vi "IMAQ FPGA Camera Link Line Builder (2 Tap U8 2X-1Y).vi"(8 "Input Valid In":bool=TRUE, 9 "Frame Valid In":bool, 10 "Line Valid In":bool, 11 "Pixel Data In":u8[](array[numeric])=[0, 0]) -> (0 "Output Valid":bool, 1 "Frame Valid Out":bool, 2 "Line Valid Out":bool, 3 "Pixel Bus x8 Out":cluster{"Pixels":u8[], "DV":bool[]}, 5 "Overflow":bool)   [LabVIEW 2020]
doc: "Camera Link cameras may return pixels from different parts of the image on each pixel clock. The Line Builder takes those pixels and combines them over multiple cycles to return a Pixel Bus of 8 pixels that are adjacent to each other. \n\nThis instance expects a camera with two taps (i.e. two pixels returned on each pixel clock). The first tap represents the left half of the image and the first valid pixels from this tap is located on the left of the image (pixels 0). The next tap represents the right half of the image and the first valid pixel from this tap is located at the center of the image."
uses:
  <vilib>/visionFPGA/Basics/Camera Link Acquisition/Controls/IMAQ FPGA Camera Link Line Builder State.ctl
  <vilib>/rvi/Emulation/niFpgaSctlEmulationGetInTimedLoop.vi
  <vilib>/Utility/error.llb/Clear Errors.vi
  <vilib>/rvi/DataTransferAndStorage/Container/Common/niFpgaContainerGetUniqueNameForEmu.vi
  <vilib>/rvi/DataTransferAndStorage/Container/Common/niFpgaContainerSetEmuInfo.vi
  <vilib>/rvi/eio/common/nirviEmuReportErrorAndStop.vi
  <vilib>/rvi/DataTransferAndStorage/Container/Common/niFpgaContainerExecOnDevCompGetState.vi
  <vilib>/rvi/Emulation/niFpgaEmulationIsFPGAContextNoSignature.vi
  <vilib>/rvi/Emulation/niFpgaProcessEmulError.vi
  <vilib>/rvi/errors/nirviReportUnexpectedCaseInternalError (U32).vi
  <vilib>/rvi/Memory/Memory_Emulation/niFpgaMemoryEmulationCacheClearOnFirstRun.vi
  <vilib>/rvi/Memory/Memory_Emulation/nirvimemoryEmulationManagerCache_MakeExclusive.vi
  <vilib>/rvi/Memory/Memory_Emulation/niFpgaMemoryEmulationValidateCache.vi
  <vilib>/rvi/Memory/Memory_Emulation/nirvimemoryEmulationManagerCache_InsertValue.vi
  <vilib>/rvi/Memory/Memory_Emulation/nirvimemoryEmulationManagerCache_ReleaseExclusive.vi
  <vilib>/rvi/Memory/Memory_Emulation/nirvimemoryEmulationManagerCache_GetValue.vi
  <vilib>/rvi/Memory/Memory_Emulation/nirvimemoryEmulationManagerCache_SetValue.vi
  <vilib>/rvi/Emulation/niFpgaSctlEmulationResourceMgr.vi
  <vilib>/rvi/LocalResourceManager/LocalResourceManager.xnode
  <vilib>/rvi/DataTransferAndStorage/Container/XNode/niFpgaContainer.xnode
  <vilib>/rvi/Memory/Memory_Emulation/niFpgaMemoryEmulationRefIn.vi
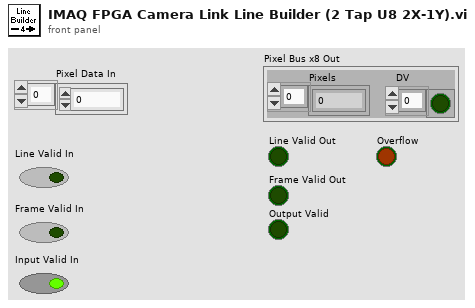
[diagram p1: front panel]
types:
  T1 = typedef "IMAQ FPGA Camera Link Line Builder State.ctl" = enum16{"Wait for First Valid Pixels", "Update Section 1", "Update Section 2", "Update Section 3", "Update Last Section", "Add Final Pack", "Add End of Line", "Check End of Image"}
  T2 = cluster{bool, u16, "Falling Edge":bool, bool, "Falling Edge":bool}
  T3 = cluster{bool, u16, "Falling Edge":bool, "Enum":T1, "Falling Edge":bool}
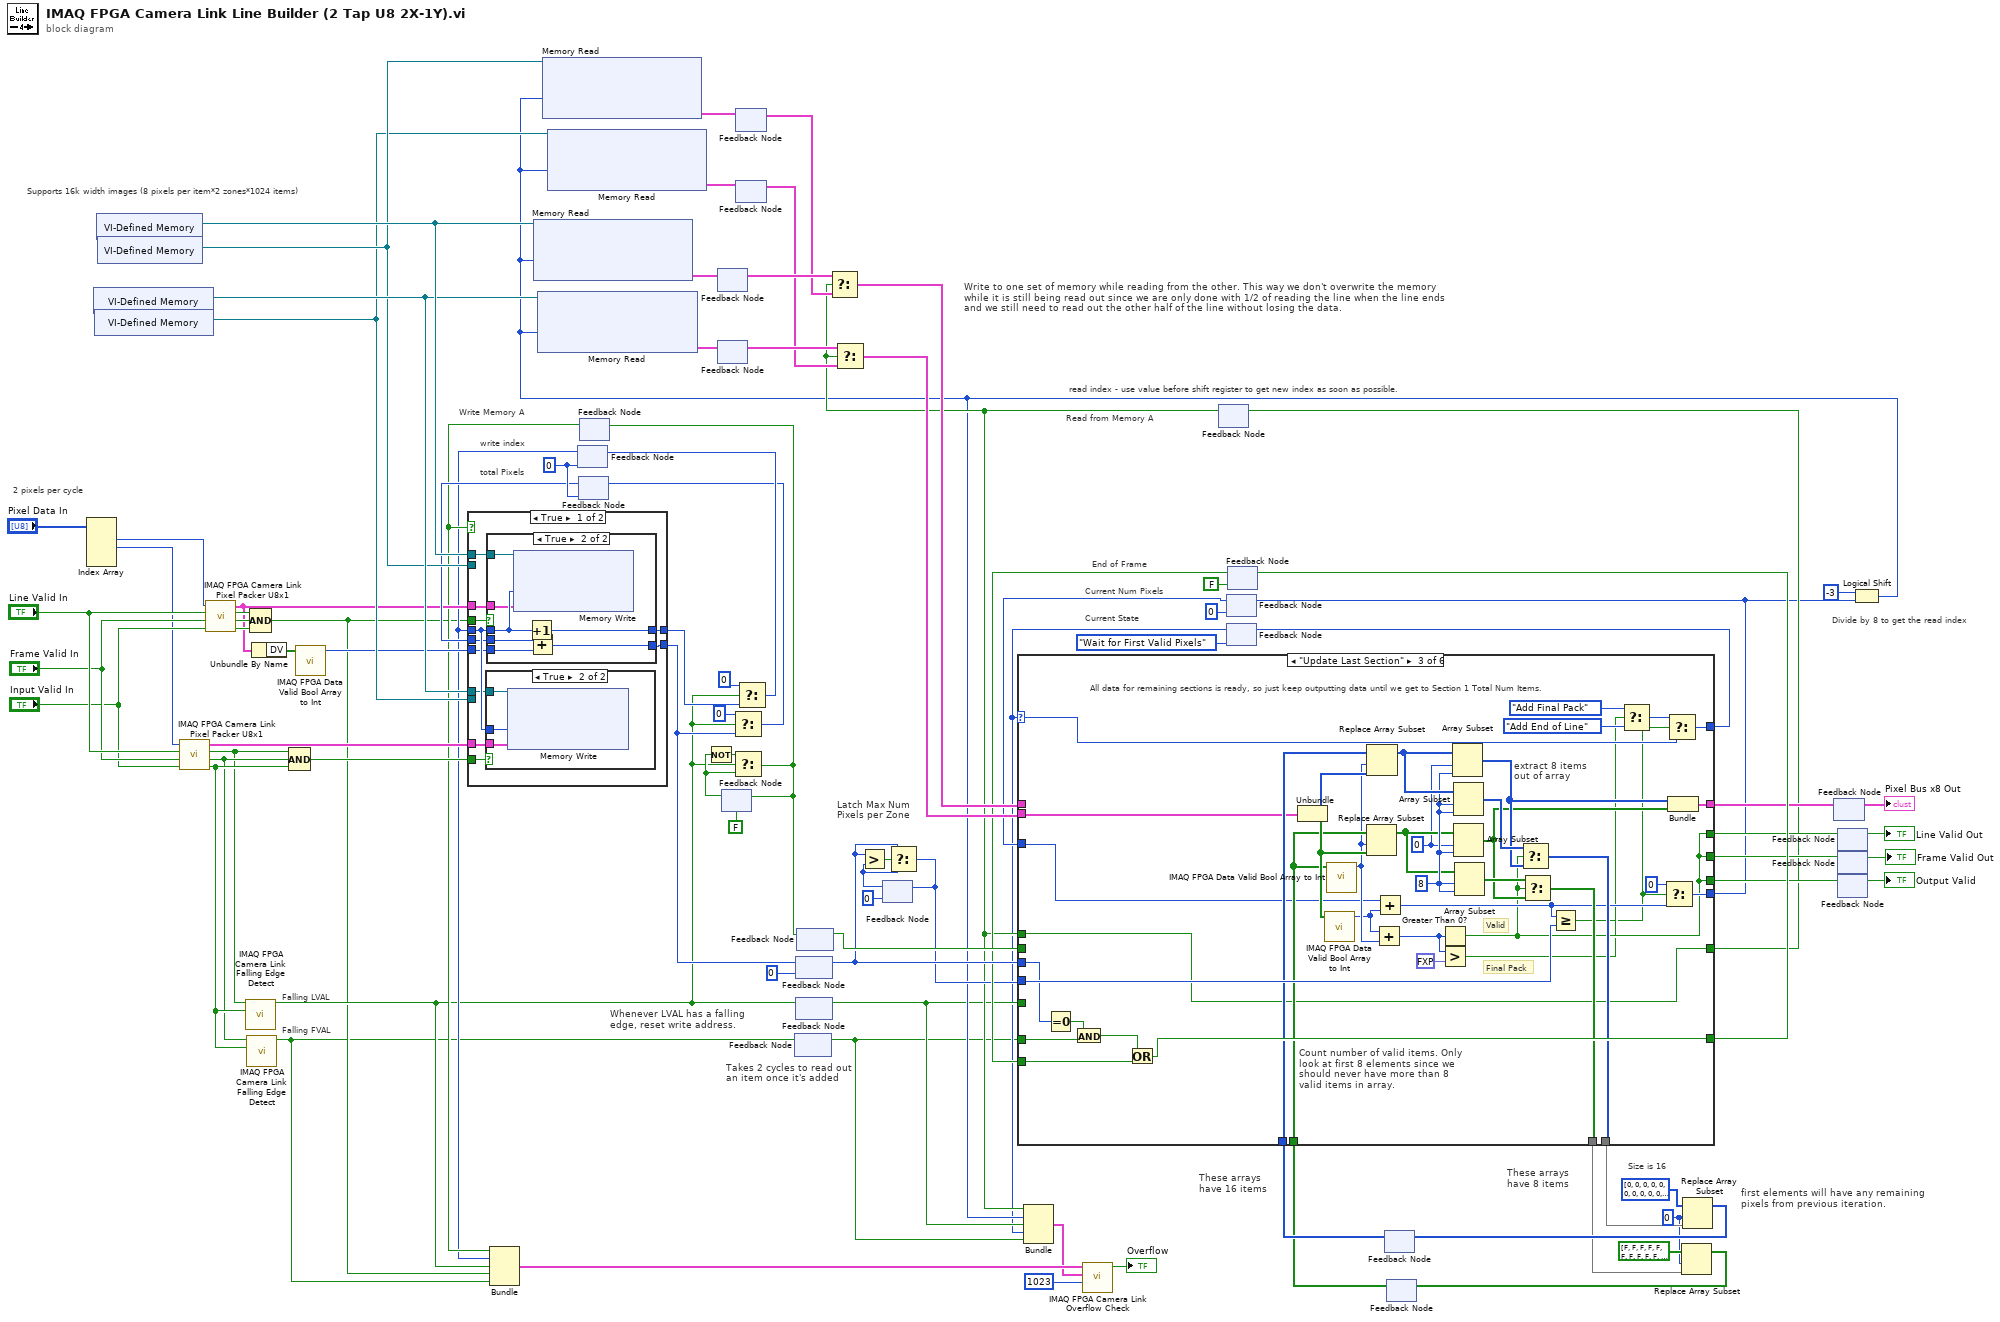
[diagram p0: block diagram]
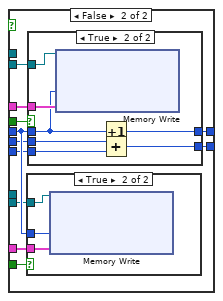
[diagram p4: hidden frame]
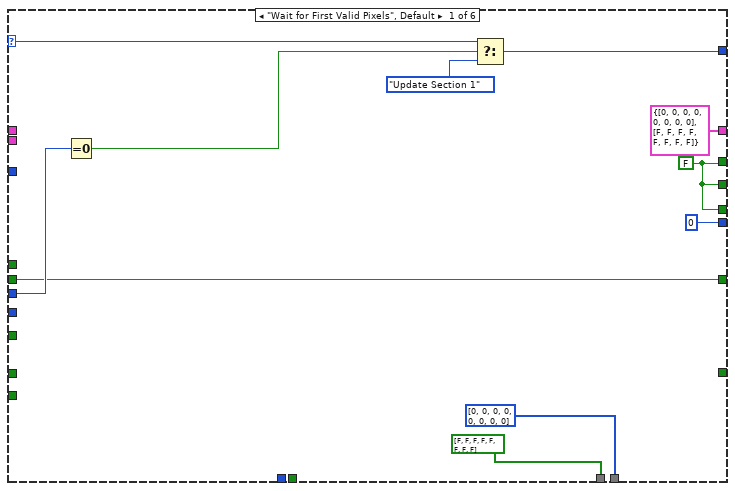
[diagram p7: hidden frame]
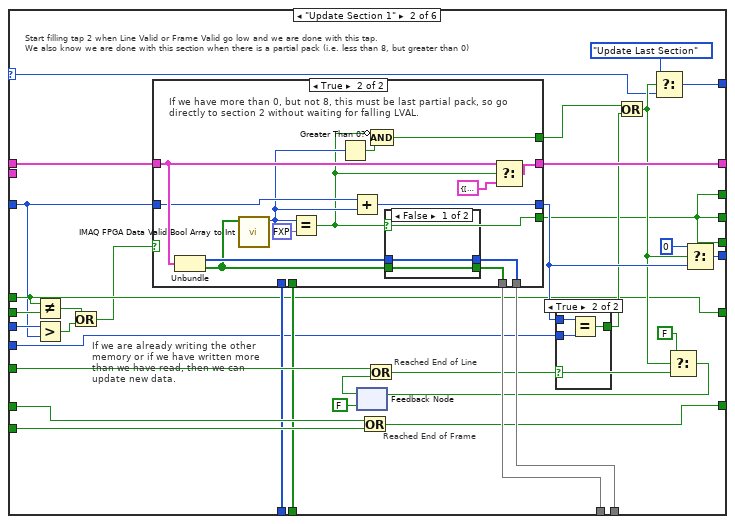
[diagram p8: hidden frame]
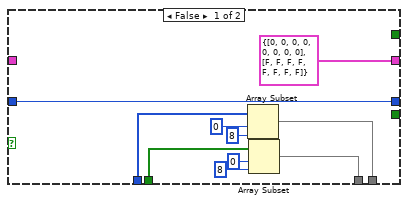
[diagram p9: hidden frame]
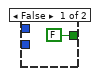
[diagram p11: hidden frame]
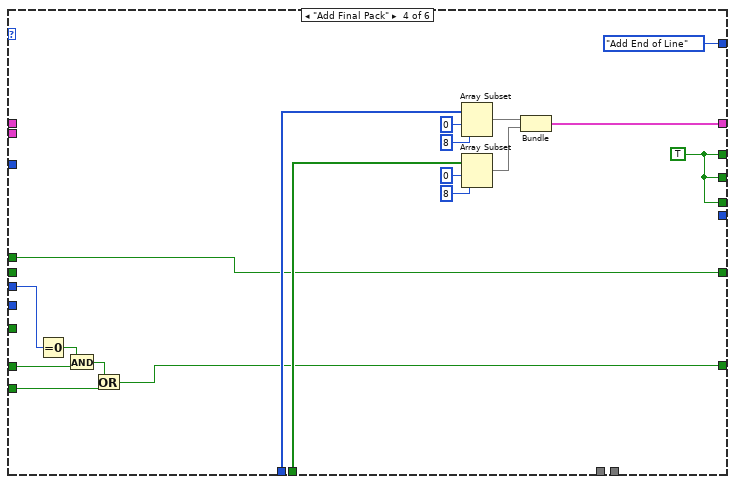
[diagram p12: hidden frame]
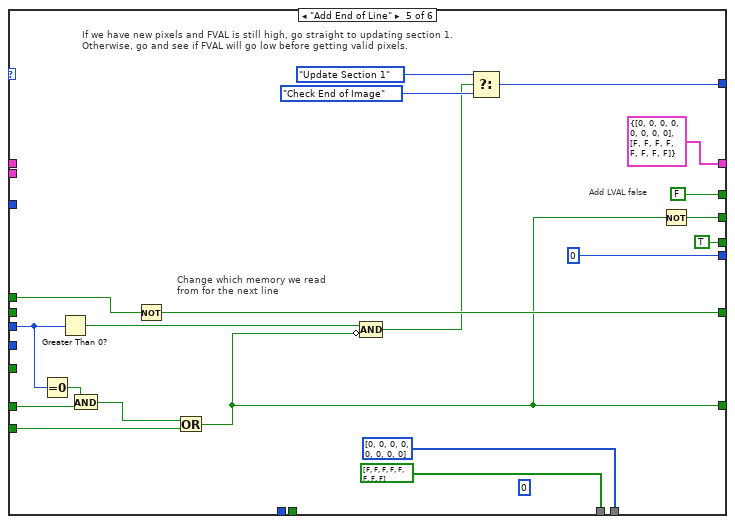
[diagram p13: hidden frame]
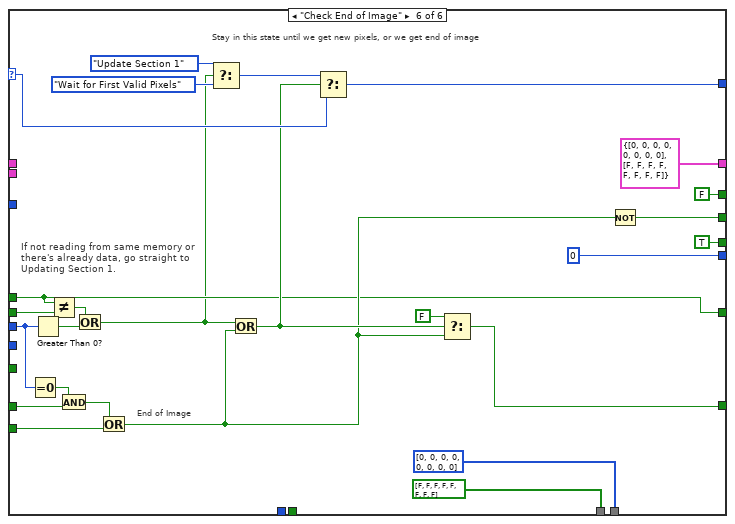
[diagram p14: hidden frame]
diagram:
  w43 = 0 ("index")
  w39 = u16 0
  # "Divide by 8 to get the read index"
  # "Latch Max Num Pixels per Zone"
  # "total Pixels"
  # "These arrays have 8 items"
  # "These arrays have 16 items"
  # "first elements will have any remaining pixels from previous iteration."
  # "Size is 16"
  # "Read from Memory A"
  # "Write Memory A"
  # "Write to one set of memory while reading from the other. This way we don't overwrite the memory while it is still being read out since we are only done with 1/2 of reading the line when the line ends and we still need to read out the other half of the line without losing the data."
  # "Falling FVAL"
  # "Falling LVAL"
  # "read index - use value before shift register to get new index as soon as possible."
  # "write index"
  # "Current State"
  # "End of Frame"
  # "Takes 2 cycles to read out an item once it's added"
  # "Current Num Pixels"
  # "Whenever LVAL has a falling edge, reset write address."
  # "Supports 16k width images (8 pixels per item*2 zones*1024 items)"
  # "2 pixels per cycle"
  n1 = Index Array(array="Pixel Data In") -> (element #1=w5:u8, element #2=w4:u8)  [unwired: 4 in, 2 out]
  n2 = xnode "VI-Defined Memory"() -> ("Memory Out"=w68:refnum<k21>)
  n3 = xnode "VI-Defined Memory"() -> ("Memory Out"=w64:refnum<k21>)
  n4 = xnode "VI-Defined Memory"() -> ("Memory Out"=w69:refnum<k21>)
  n5 = xnode "VI-Defined Memory"() -> ("Memory Out"=w65:refnum<k21>)
  n6 = call <vilib>:"IMAQ FPGA Camera Link Pixel Packer U8x1.vi"("Input Valid"="Input Valid In", "Frame Valid In"="Frame Valid In", "Line Valid In"="Line Valid In", "Pixel In"=w4) -> ("Output Valid"=w3:bool, "Frame Valid Out"=w2:bool, "Line Valid Out"=w1:bool, "Pixel Bus x8 Out"=w57:cluster{"Pixels":u8[], "DV":bool[]})  [unwired: 4 in]
  n7 = call <vilib>:"IMAQ FPGA Camera Link Pixel Packer U8x1.vi"("Input Valid"="Input Valid In", "Frame Valid In"="Frame Valid In", "Line Valid In"="Line Valid In", "Pixel In"=w5) -> ("Output Valid"=w83:bool, "Frame Valid Out"=w84:bool, "Line Valid Out"=w85:bool, "Pixel Bus x8 Out"=w33:cluster{"Pixels":u8[], "DV":bool[]})  [unwired: 4 in]
  n8 = call <vilib>:"IMAQ FPGA Camera Link Falling Edge Detect.vi"("Input Valid"=w3, "Input"=w1) -> ("Falling Edge"=w17:bool)  [unwired: 9 in]
  n9 = call <vilib>:"IMAQ FPGA Camera Link Falling Edge Detect.vi"("Input Valid"=w3, "Input"=w2) -> ("Falling Edge"=w15:bool)  [unwired: 9 in]
  n10 = Compound Arithmetic op=AND(w85, w84, w83) -> (w16:bool)
  n11 = Unbundle By Name(w33) -> ("DV"=w42:bool[])
  n12 = Compound Arithmetic op=AND(w1, w2, w3) -> (w55:bool)
  n13 = call <vilib>:"IMAQ FPGA Data Valid Bool Array to Int.vi"("DV In"=w42) -> ("Sum DV Out"=w37:u8)  [unwired: 10 in]
  n14 = feedback #1(w39) -> (w18:u16)
  n15 = feedback #2(w39) -> (w38:u16)
  n16 = feedback #3() -> (w19:bool)  [unwired: 1 in]
  n17 = case shown="True" w19 {
    tunnel: [w102 w125] -> w86
    tunnel: w18 -> [w101 w124]
    tunnel: w16 -> [w96 w123]
    tunnel: w33 -> [w100 w122]
    tunnel: w57 -> [w99 w121]
    tunnel: w69 -> [w98 _]
    tunnel: w68 -> [w97 _]
    tunnel: w65 -> [_ w120]
    tunnel: w64 -> [_ w119]
    tunnel: w55 -> [w95 w118]
    tunnel: [w94 w117] -> w36
    tunnel: w38 -> [w93 w116]
    tunnel: w37 -> [w92 w115]
    frame True {
      n18 = case shown="True" w95 {
        tunnel: w99 -> [_ w104]
        tunnel: w97 -> [_ w105]
        tunnel: w101 -> [_ w103]
        frame False {
        }
        frame True {
          n19 = xnode ("Memory Write")("Address"=w103, "Data"=w104, "Memory In"=w105) -> ()  [unwired: 1 out]
        }
      }
      n20 = case shown="True" w96 {
        tunnel: [w106 w108] -> w102
        tunnel: w101 -> [w107 w113]
        tunnel: w98 -> [_ w114]
        tunnel: w100 -> [_ w112]
        tunnel: [w107 w111] -> w94
        tunnel: w93 -> [w106 w110]
        tunnel: w92 -> [_ w109]
        frame False {
        }
        frame True {
          n21 = xnode ("Memory Write")("Address"=w113, "Data"=w112, "Memory In"=w114) -> ()  [unwired: 1 out]
          n22 = Increment(x=w113) -> (x+1=w111:u16)
          n23 = Add(x=w110, y=w109) -> (x+y=w108:u16)
        }
      }
    }
    frame False {
      n24 = case shown="True" w118 {
        tunnel: w121 -> [_ w127]
        tunnel: w119 -> [_ w128]
        tunnel: w124 -> [_ w126]
        frame False {
        }
        frame True {
          n25 = xnode ("Memory Write")("Address"=w126, "Data"=w127, "Memory In"=w128) -> ()  [unwired: 1 out]
        }
      }
      n26 = case shown="True" w123 {
        tunnel: [w129 w133] -> w125
        tunnel: w124 -> [w130 w135]
        tunnel: w120 -> [_ w137]
        tunnel: w122 -> [_ w136]
        tunnel: [w130 w134] -> w117
        tunnel: w116 -> [w129 w132]
        tunnel: w115 -> [_ w131]
        frame False {
        }
        frame True {
          n27 = xnode ("Memory Write")("Address"=w135, "Data"=w136, "Memory In"=w137) -> ()  [unwired: 1 out]
          n28 = Increment(x=w135) -> (x+1=w134:u16)
          n29 = Add(x=w132, y=w131) -> (x+y=w133:u16)
        }
      }
    }
  }
  n30 = Bundle(w19, w18, "Falling Edge"=w17, w16, "Falling Edge"=w15) -> (w14:T2)  [unwired: 1 in]
  n31 = feedback #4() -> (w61:cluster{"Pixels":u8[], "DV":bool[]})  [unwired: 1 in]
  n32 = feedback #5() -> (w59:cluster{"Pixels":u8[], "DV":bool[]})  [unwired: 1 in]
  n33 = feedback #6(FALSE) -> (w41:bool)
  n34 = Not(x=w41) -> (.not. x?=w81:bool)
  n35 = Select(t=u16 0, s=w17, f=w86) -> (s? t:f=w34:u16)
  n36 = feedback-in #2(w34) -> ()
  n37 = Select(t=w81, s=w17, f=w41) -> (s? t:f=w32:bool)
  n38 = feedback-in #3(w32) -> ()
  n39 = feedback-in #6(w32) -> ()
  n40 = feedback #7() -> (w60:cluster{"Pixels":u8[], "DV":bool[]})  [unwired: 1 in]
  n41 = feedback #8() -> (w58:cluster{"Pixels":u8[], "DV":bool[]})  [unwired: 1 in]
  n42 = Select(t=u16 0, s=w17, f=w36) -> (s? t:f=w35:u16)
  n43 = feedback-in #1(w35) -> ()
  n44 = feedback #9() -> (w8:bool)  [unwired: 1 in]
  n45 = feedback-in #9(w15) -> ()
  n46 = feedback-in #10(w86) -> ()
  n47 = feedback #10(u16 0) -> (w30:u16)
  n48 = feedback-in #11(w17) -> ()
  n49 = feedback #11() -> (w11:bool)  [unwired: 1 in]
  n50 = feedback #12() -> (w47:bool)  [unwired: 1 in]
  n51 = feedback-in #12(w32) -> ()
  n52 = feedback #13(u16 0) -> (w29:u16)
  n53 = Greater?(x=w30, y=w29) -> (0:w31:bool)
  n54 = Select(t=w30, s=w31, f=w29) -> (s? t:f=w20:u16)
  n55 = feedback-in #13(w20) -> ()
  n56 = feedback #14() -> (w13:bool)  [unwired: 1 in]
  n57 = Select(t=w61, s=w13, f=w60) -> (s? t:f=w46:cluster{"Pixels":u8[], "DV":bool[]})
  n58 = Select(t=w59, s=w13, f=w58) -> (s? t:f=w56:cluster{"Pixels":u8[], "DV":bool[]})
  n59 = feedback #15(u16 0) -> (w22:u16)
  n60 = feedback #16(IMAQ_FPGA_Camera_Link_Line_Builder_State."Wait for First Valid Pixels" ("Enum")) -> (w9:T1)
  n61 = feedback #17(FALSE) -> (w24:bool)
  n62 = feedback #18() -> (w45:u8[])  [unwired: 1 in]
  n63 = feedback #19() -> (w44:bool[])  [unwired: 1 in]
  n64 = case shown="\"Update Last Section\"" w9 {
    selector: w9 -> [w148 w149 w239 _ _ w309]
    tunnel: [w147 w181 w251 IMAQ_FPGA_Camera_Link_Line_Builder_State."Add End of Line" ("Enum") w284 w310] -> w21
    tunnel: w11 -> [_ w179 _ _ _ _]
    tunnel: w8 -> [_ w175 w221 w253 w273 w296]
    tunnel: [u16 0 w178 w247 _ u16 0 u16 0] -> w27
    tunnel: w22 -> [_ w155 w228 _ _ _]
    tunnel: w30 -> [w143 w156 w222 w254 w274 w297]
    tunnel: w20 -> [_ w168 w248 _ _ _]
    tunnel: [_ w171 w249 w256 w270 w306] -> w87
    tunnel: w24 -> [_ w176 w250 w257 w288 w312]
    tunnel: w46 -> [_ w165 _ _ _ _]
    tunnel: w56 -> [_ _ w214 _ _ _]
    tunnel: w47 -> [w142 w158 _ _ _ w293]
    tunnel: [w142 w159 w216 w258 w279 w292] -> w48
    tunnel: w13 -> [_ w159 w216 w258 w280 w292]
    tunnel: w44 -> [_ w169 w238 w261 _ _]
    tunnel: w45 -> [_ w170 w243 w262 _ _]
    tunnel: [cluster{"Pixels":u8[], "DV":bool[]} {"Pixels"=[0, 0, 0, 0, 0, 0, 0, 0], "DV"=[FALSE, FALSE, FALSE, FALSE, FALSE, FALSE, FALSE, FALSE]} ("Data") w174 w246 w260 cluster{"Pixels":u8[], "DV":bool[]} {"Pixels"=[0, 0, 0, 0, 0, 0, 0, 0], "DV"=[FALSE, FALSE, FALSE, FALSE, FALSE, FALSE, FALSE, FALSE]} ("Data") cluster{"Pixels":u8[], "DV":bool[]} {"Pixels"=[0, 0, 0, 0, 0, 0, 0, 0], "DV"=[FALSE, FALSE, FALSE, FALSE, FALSE, FALSE, FALSE, FALSE]} ("Data")] -> w77
    tunnel: [w138 w152 w219 w259 FALSE FALSE] -> w75
    tunnel: [w138 w152 w219 w259 w281 w302] -> w74
    tunnel: [w138 w152 w219 w259 TRUE TRUE] -> w73
    tunnel: [bool[] [FALSE, FALSE, FALSE, FALSE, FALSE, FALSE, FALSE, FALSE] ("DV") w173 w232 _ bool[] [FALSE, FALSE, FALSE, FALSE, FALSE, FALSE, FALSE, FALSE] bool[] [FALSE, FALSE, FALSE, FALSE, FALSE, FALSE, FALSE, FALSE]] -> w49
    tunnel: [u8[] [0, 0, 0, 0, 0, 0, 0, 0] ("Pixels") w172 w231 _ u8[] [0, 0, 0, 0, 0, 0, 0, 0] ("Pixels") u8[] [0, 0, 0, 0, 0, 0, 0, 0] ("Pixels")] -> w50
    frame "Wait for First Valid Pixels", Default {
      w138 = FALSE
      n65 = Equal To 0?(x=w143) -> (x = 0?=w146:bool)
      n66 = Select(t=w148, s=w146, f=IMAQ_FPGA_Camera_Link_Line_Builder_State."Update Section 1") -> (s? t:f=w147:T1)
    }
    frame "Update Section 1" {
      # "If we are already writing the other memory or if we have written more than we have read, then we can update new data."
      # "Reached End of Frame"
      # "Reached End of Line"
      # "Start filling tap 2 when Line Valid or Frame Valid go low and we are done with this tap.\nWe also know we are done with this section when there is a partial pack (i.e. less than 8, but greater than 0)"
      n67 = Not Equal?(x=w159, y=w158) -> (x != y?=w157:bool)
      n68 = Greater?(x=w156, y=w155) -> (0:w154:bool)
      n69 = Or(x=w157, y=w154) -> (x .or. y?=w153:bool)
      n70 = case shown="True" w153 {
        tunnel: w165 -> [_ w202]
        tunnel: w155 -> [w191 w200]
        tunnel: [w191 w205] -> w177
        tunnel: [cluster{"Pixels":u8[], bool[]} {"Pixels"=[0, 0, 0, 0, 0, 0, 0, 0], [FALSE, FALSE, FALSE, FALSE, FALSE, FALSE, FALSE, FALSE]} w204] -> w174
        tunnel: [w182 w195] -> w173
        tunnel: [w186 w196] -> w172
        tunnel: w170 -> [w189 _]
        tunnel: w169 -> [w185 _]
        tunnel: [_ w194] -> w152
        tunnel: [_ w192] -> w151
        frame False {
          n71 = Array Subset(array=w189, index=0, length=8) -> (w186:u8[])
          n72 = Array Subset(array=w185, index=0, length=8) -> (w182:bool[])
        }
        frame True {
          # "If we have more than 0, but not 8, this must be last partial pack, so go directly to section 2 without waiting for falling LVAL."
          n73 = Unbundle(w202) -> ("Pixels"=w198:u8[], "DV"=w197:bool[])
          n74 = call <vilib>:"IMAQ FPGA Data Valid Bool Array to Int.vi"("DV In"=w197) -> ("Sum DV Out"=w199:u8)  [unwired: 10 in]
          n75 = Equal?(x=w199, y=fxp<+,4,4> 8.0) -> (x = y?=w194:bool)
          n76 = Greater Than 0?(x=w199) -> (x > 0?=w193:bool)
          n77 = Add(x=w200, y=w199) -> (x+y=w205:u16)
          n78 = Compound Arithmetic op=AND(invert w194, w193) -> (w192:bool)
          n79 = case shown="False" w194 {
            tunnel: w198 -> [w207 _]
            tunnel: w197 -> [w206 _]
            tunnel: [w207 _] -> w196
            tunnel: [w206 _] -> w195
            frame False {
            }
            frame True {
            }
          }
          n80 = Select(t=w202, s=w194, f=cluster{"Pixels":u8[], "DV":bool[]} {"Pixels"=[0, 0, 0, 0, 0, 0, 0, 0], "DV"=[FALSE, FALSE, FALSE, FALSE, FALSE, FALSE, FALSE, FALSE]}) -> (s? t:f=w204:cluster{"Pixels":u8[], "DV":bool[]})
        }
      }
      n81 = feedback #20(FALSE) -> (w164:bool)
      n82 = Or(x=w175, y=w176) -> (x .or. y?=w171:bool)
      n83 = Or(x=w179, y=w164) -> (x .or. y?=w163:bool)
      n84 = case shown="True" w163 {
        tunnel: w168 -> [_ w210]
        tunnel: w177 -> [_ w211]
        tunnel: [FALSE w209] -> w166
        frame False {
        }
        frame True {
          n85 = Equal?(x=w211, y=w210) -> (x = y?=w209:bool)
        }
      }
      n86 = Or(x=w151, y=w166) -> (x .or. y?=w162:bool)
      n87 = Select(t=IMAQ_FPGA_Camera_Link_Line_Builder_State."Update Last Section" ("Enum"), s=w162, f=w149) -> (s? t:f=w181:T1)
      n88 = Select(t=FALSE, s=w162, f=w163) -> (s? t:f=w160:bool)
      n89 = feedback-in #20(w160) -> ()
      n90 = Select(t=u16 0, s=w162, f=w177) -> (s? t:f=w178:u16)
    }
    frame "Update Last Section" {
      w230 = 0 ("index")
      w241 = 8 ("length")
      # "Final Pack"
      # "Valid"
      # "extract 8 items out of array"
      # "Count number of valid items. Only look at first 8 elements since we should never have more than 8 valid items in array."
      # "All data for remaining sections is ready, so just keep outputting data until we get to Section 1 Total Num Items."
      n91 = Equal To 0?(x=w222) -> (x = 0?=w223:bool)
      n92 = And(x=w223, y=w221) -> (x .and. y?=w220:bool)
      n93 = Or(x=w220, y=w250) -> (x .or. y?=w249:bool)
      n94 = Unbundle(w214) -> ("Pixels"=w245:u8[], "DV"=w244:bool[])
      n95 = call <vilib>:"IMAQ FPGA Data Valid Bool Array to Int.vi"("DV In"=w244) -> ("Sum DV Out"=w227:u8)  [unwired: 10 in]
      n96 = call <vilib>:"IMAQ FPGA Data Valid Bool Array to Int.vi"("DV In"=w238) -> ("Sum DV Out"=w237:u8)  [unwired: 10 in]
      n97 = Replace Array Subset(array=w238, new element=w244, index=w237) -> (w240:bool[])
      n98 = Replace Array Subset(array=w243, new element=w245, index=w237) -> (w242:u8[])
      n99 = Add(x=w227, y=w237) -> (x+y=w217:u8)
      n100 = Add(x=w228, y=w227) -> (x+y=w229:u16)
      n101 = Greater Than 0?(x=w217) -> (x > 0?=w219:bool)
      n102 = Greater?(x=w217, y=fxp<+,5,5> 8.0) -> (0:w218:bool)
      n103 = Array Subset(array=w242, index=w230, length=w241) -> (w235:u8[])
      n104 = Array Subset(array=w242, index=w241, length=w241) -> (w236:u8[])
      n105 = Array Subset(array=w240, index=w230, length=w241) -> (w233:bool[])
      n106 = Array Subset(array=w240, index=w241, length=w241) -> (w234:bool[])
      n107 = Select(t=w236, s=w219, f=w235) -> (s? t:f=w231:u8[])
      n108 = Select(t=w234, s=w219, f=w233) -> (s? t:f=w232:bool[])
      n109 = Greater Or Equal?(x=w229, y=w248) -> (x >= y?=w212:bool)
      n110 = Select(t=IMAQ_FPGA_Camera_Link_Line_Builder_State."Add Final Pack", s=w218, f=IMAQ_FPGA_Camera_Link_Line_Builder_State."Add End of Line" ("t")) -> (s? t:f=w225:T1)
      n111 = Select(t=u16 0, s=w212, f=w229) -> (s? t:f=w247:u16)
      n112 = Select(t=w225, s=w212, f=w239) -> (s? t:f=w251:T1)
      n113 = Bundle(w235, w233) -> (w246:cluster{u8[], bool[]})  [unwired: 1 in]
    }
    frame "Add Final Pack" {
      w259 = TRUE
      n114 = Equal To 0?(x=w254) -> (x = 0?=w255:bool)
      n115 = And(x=w255, y=w253) -> (x .and. y?=w252:bool)
      n116 = Or(x=w252, y=w257) -> (x .or. y?=w256:bool)
      n117 = Array Subset(array=w262, index=0, length=8) -> (w264:u8[])
      n118 = Array Subset(array=w261, index=0, length=8) -> (w263:bool[])
      n119 = Bundle(w264, w263) -> (w260:cluster{u8[], bool[]})  [unwired: 1 in]
    }
    frame "Add End of Line" {
      (unwired) i8 0
      # "Change which memory we read from for the next line"
      # "Add LVAL false"
      # "If we have new pixels and FVAL is still high, go straight to updating section 1. Otherwise, go and see if FVAL will go low before getting valid pixels."
      n120 = Equal To 0?(x=w274) -> (x = 0?=w275:bool)
      n121 = Greater Than 0?(x=w274) -> (x > 0?=w287:bool)
      n122 = And(x=w275, y=w273) -> (x .and. y?=w272:bool)
      n123 = Not(x=w280) -> (.not. x?=w279:bool)
      n124 = Or(x=w272, y=w288) -> (x .or. y?=w270:bool)
      n125 = Compound Arithmetic op=AND(w287, invert w270) -> (w271:bool)
      n126 = Select(t=IMAQ_FPGA_Camera_Link_Line_Builder_State."Update Section 1" ("Enum"), s=w271, f=IMAQ_FPGA_Camera_Link_Line_Builder_State."Check End of Image" ("Enum")) -> (s? t:f=w284:T1)
      n127 = Not(x=w270) -> (.not. x?=w281:bool)
    }
    frame "Check End of Image" {
      # "If not reading from same memory or there's already data, go straight to Updating Section 1."
      # "Stay in this state until we get new pixels, or we get end of image"
      # "End of Image"
      n128 = Equal To 0?(x=w297) -> (x = 0?=w298:bool)
      n129 = Greater Than 0?(x=w297) -> (x > 0?=w294:bool)
      n130 = Not Equal?(x=w292, y=w293) -> (x != y?=w291:bool)
      n131 = And(x=w298, y=w296) -> (x .and. y?=w295:bool)
      n132 = Or(x=w291, y=w294) -> (x .or. y?=w290:bool)
      n133 = Or(x=w295, y=w312) -> (x .or. y?=w303:bool)
      n134 = Select(t=IMAQ_FPGA_Camera_Link_Line_Builder_State."Update Section 1" ("Enum"), s=w290, f=IMAQ_FPGA_Camera_Link_Line_Builder_State."Wait for First Valid Pixels" ("Enum")) -> (s? t:f=w311:T1)
      n135 = Or(x=w290, y=w303) -> (x .or. y?=w308:bool)
      n136 = Select(t=w311, s=w308, f=w309) -> (s? t:f=w310:T1)
      n137 = Select(t=FALSE, s=w308, f=w303) -> (s? t:f=w306:bool)
      n138 = Not(x=w303) -> (.not. x?=w302:bool)
    }
  }
  n139 = feedback-in #14(w48) -> ()
  n140 = feedback-in #15(w27) -> ()
  n141 = feedback-in #16(w21) -> ()
  n142 = feedback-in #17(w87) -> ()
  n143 = Replace Array Subset(array=bool[] [FALSE, FALSE, FALSE, FALSE, FALSE, FALSE, FALSE, FALSE, FALSE, FALSE, FALSE, FALSE, FALSE, FALSE, FALSE, FALSE], new element=w49, index=w43) -> (w51:bool[])
  n144 = feedback-in #19(w51) -> ()
  n145 = Replace Array Subset(array=u8[] [0, 0, 0, 0, 0, 0, 0, 0, 0, 0, 0, 0, 0, 0, 0, 0] ("Pixels"), new element=w50, index=w43) -> (w53:u8[])
  n146 = feedback-in #18(w53) -> ()
  n147 = feedback #21() -> (→"Pixel Bus x8 Out":cluster{"Pixels":u8[], "DV":bool[]})  [unwired: 1 in]
  n148 = feedback-in #21(w77) -> ()
  n149 = feedback #22() -> (→"Line Valid Out":bool)  [unwired: 1 in]
  n150 = feedback-in #22(w75) -> ()
  n151 = feedback #23() -> (→"Frame Valid Out":bool)  [unwired: 1 in]
  n152 = feedback-in #23(w74) -> ()
  n153 = feedback #24() -> (→"Output Valid":bool)  [unwired: 1 in]
  n154 = feedback-in #24(w73) -> ()
  n155 = Logical Shift(y=i16 -3, x=w27) -> (x << y=w12:u16)
  n156 = xnode ("Memory Read")("Address"=w12, "Memory In"=w69) -> ("Data"=w67:cluster{"Pixels":u8[], "DV":bool[]})  [unwired: 1 out]
  n157 = xnode ("Memory Read")("Address"=w12, "Memory In"=w68) -> ("Data"=w66:cluster{"Pixels":u8[], "DV":bool[]})  [unwired: 1 out]
  n158 = xnode ("Memory Read")("Address"=w12, "Memory In"=w65) -> ("Data"=w62:cluster{"Pixels":u8[], "DV":bool[]})  [unwired: 1 out]
  n159 = xnode ("Memory Read")("Address"=w12, "Memory In"=w64) -> ("Data"=w63:cluster{"Pixels":u8[], "DV":bool[]})  [unwired: 1 out]
  n160 = feedback-in #4(w67) -> ()
  n161 = feedback-in #5(w66) -> ()
  n162 = feedback-in #7(w62) -> ()
  n163 = feedback-in #8(w63) -> ()
  n164 = Bundle(w13, w12, "Falling Edge"=w11, "Enum"=w9, "Falling Edge"=w8) -> (w10:T3)  [unwired: 1 in]
  n165 = call <vilib>:"IMAQ FPGA Camera Link Overflow Check.vi"("Max Index"=u16 1023, "Read Info"=w10, "Write Info"=w14) -> ("Overlfow"=→"Overflow":bool)  [unwired: 8 in]
